vi "Test Get Summary of Compare 2D Array.vi"(8 "error in (no error)":errorcluster, 11 "Result Model Result Recording Test in":refnum<class "Result Model Result Recording Test.lvclass">) -> (0 "error out":errorcluster, 3 "Result Model Result Recording Test out":refnum<class "Result Model Result Recording Test.lvclass">)   [LabVIEW 2020, in "Result Model Result Recording Test.lvclass"]
uses:
  Result Model Result Recording Test.lvclass
  C:/Program Files (x86)/National Instruments/LabVIEW 2020/vi.lib/Astemes/LUnit/Core/LUnit Test Case/Test Case.lvclass
  source/Core/Result/Result.ctl
  source/Core/Result/Status.ctl
  source/Core/Result/Type.ctl
  <vilib>/Astemes/LUnit/Core/LUnit Test Case/Test Case.lvclass/Test Case.ctl
  865a11a4-746d-41de-93c1-4db6b0010296.vi
  <vilib>/Astemes/LUnit/Core/LUnit Test Case/Private/Append Pass Result.vi
  <vilib>/Astemes/LUnit/Core/LUnit Test Case/Private/Append Fail Result.vi
  865a11a4-746d-41de-93c1-4db6b0010296.vi/9c5d11cd-9439-4240-a1ee-d9baace9c924.vi
  <vilib>/Astemes/LUnit/Core/LUnit Test Case/Private/Run In UI.vi
  <vilib>/Utility/error.llb/Clear Errors.vi
  source/User Interface/Result Model by Reference/Result Model by Reference.lvclass
  source/Core/Result/Result.lvlib
panel:
  out "Summary":string
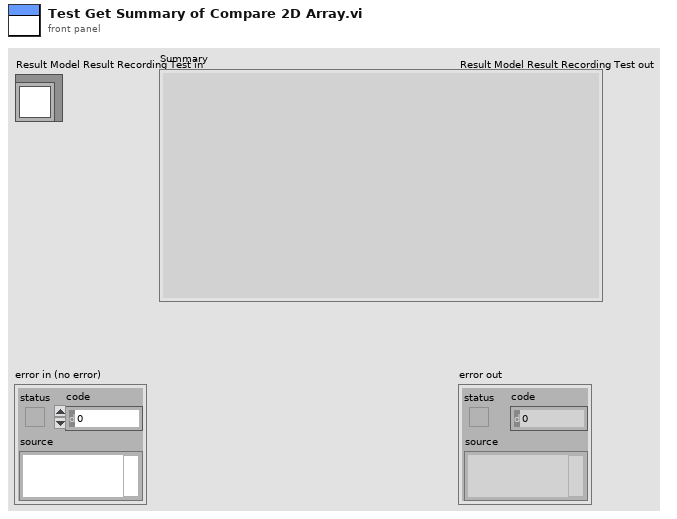
[diagram p1: front panel]
types:
  T1 = typedef "Result.lvlib/Result.ctl" = cluster{"Name":string, "Description":string, "Status":T2, "Result Type":T3, "Execution Time":dbl, "Data":cluster{"Expected":variant, "Actual":variant, "Delta":variant}}
  T2 = typedef "Result.lvlib/Status.ctl" = enum16{"", "Passed", "Failed", "Error", "Skipped", "Setup Error", "Broken", "Teardown Error"}
  T3 = typedef "Result.lvlib/Type.ctl" = enum16{"Test Case", "Test Suite", "Test Run", "Pass", "Fail", "Skip", "Pass if", "Fail if", "Pass if Error", "Fail if Error", "Pass if Equal", "Fail if Equal"}
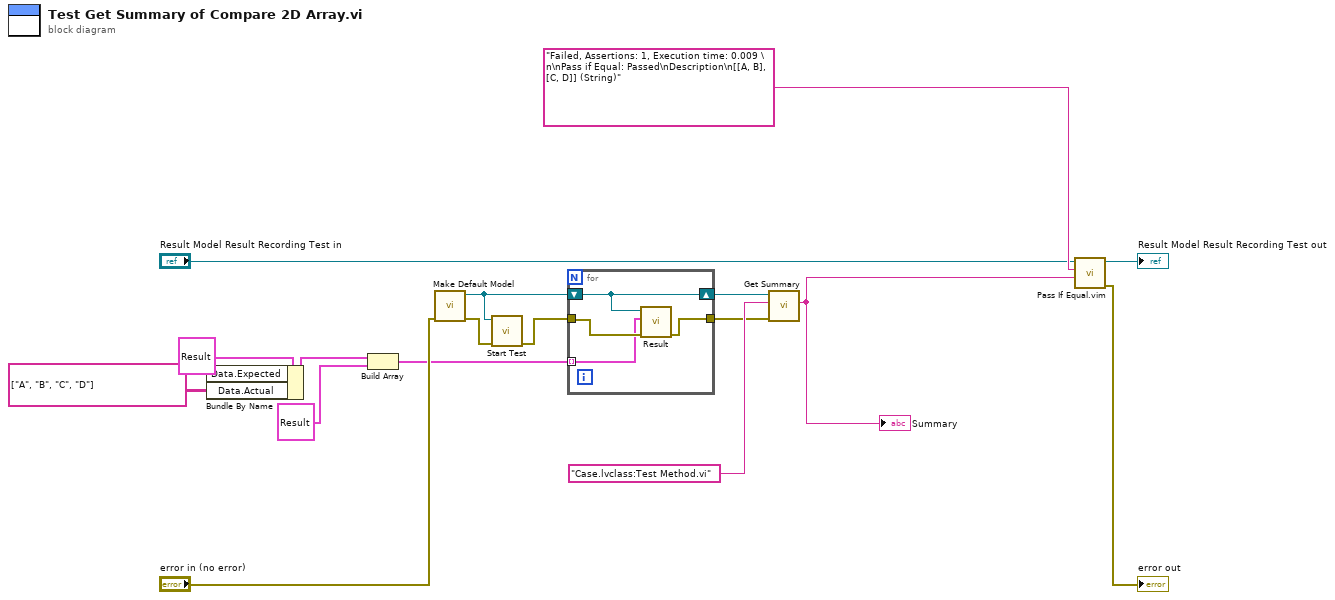
[diagram p0: block diagram]
diagram:
  w1 = string[][] [["A", "B"], ["C", "D"]]
  n1 = Bundle By Name(cluster=T1 {"Name"="Case.lvclass:Test Method.vi", "Description"="Description", "Status"=enum."Passed", "Result Type"=enum."Pass if Equal", "Execution Time"=0.0, "Data"={"Expected"=variant, "Actual"=variant, "Delta"=variant}} ("Result"), "Data.Expected"=w1, "Data.Actual"=w1) -> (w2:T1)
  n2 = Build Array(w2, T1 {"Name"="Case.lvclass:Test Method.vi", "Description"="", "Status"=enum."Failed", "Result Type"=enum."Test Case", "Execution Time"=0.009, "Data"={"Expected"=variant, "Actual"=variant, "Delta"=variant}} ("Result")) -> (w3:T1[])
  n3 = call "Make Default Model.vi"("error in (no error)"="error in (no error)") -> ("error out"=w9:errorcluster, "Result Model out"=w7:refnum<class "Result Model by Reference.lvclass">)  [unwired: 9 in]
  n4 = call "Start Test.vi"("error in (no error)"=w9, "Result Model In"=w7) -> ("error out"=w8:errorcluster)  [unwired: 9 in]
  n5 = for {
    shift-right: [w20] -> w14
    shift-left: w7 -> [w20]
    tunnel: w8 -> [w21]
    tunnel: [w19] -> w6
    tunnel: w3 -> [w18] mode=indexing
    n6 = call-dynamic "Result.vi"("error in (no error)"=w21, "Results"=w18, "Result Model by Reference In"=w20) -> ("error out"=w19:errorcluster)  [unwired: 8 in]
  }
  n7 = call "Get Summary.vi"("error in (no error)"=w6, "Item"="Case.lvclass:Test Method.vi", "Result Model by Reference In"=w14) -> ("Summary"=w12:string)  [unwired: 7 in, 1 out]
  "Summary" <- w12
  n8 = call "Pass If Equal.vim"("Actual"=w12, "Expected"="Failed, Assertions: 1, Execution time: 0.009 \n\nPass if Equal: Passed\nDescription\n[[A, B], [C, D]] (String)", "LUnit Test Case In"="Result Model Result Recording Test in") -> ("error out"=→"error out":errorcluster, "LUnit Test Case Out"=→"Result Model Result Recording Test out":refnum<class "Result Model Result Recording Test.lvclass">)  [unwired: 7 in]
